vi "Test Bench v21 - TDMS.vi"() -> ()   [LabVIEW 2022 SP3]
doc: "Use this template to build a producer/consumer design pattern. Use this template when you need to execute a process, such as data analysis, when a data source, such as a triggered acquisition, produces data at an uneven rate and you need to execute the process when the data becomes available."
uses:
  WhiteNoise.ctl
  <vilib>/Utility/error.llb/DialogType.ctl
  <vilib>/Platform/TimedLoop/XDataNode/timing_clust.ctl
  <vilib>/Platform/TimedLoop/XDataNode/nitl_modes.ctl
  <vilib>/Platform/TimedLoop/XDataNode/wakeup.ctl
  <vilib>/DAQmx/write.llb/DAQmx Write (Analog Wfm 1Chan NSamp).vi
  <vilib>/DAQmx/read.llb/DAQmx Read (Analog Wfm 1Chan NSamp).vi
  <vilib>/DAQmx/miscellaneous.llb/DAQmx Fill In Error Info.vi
  <vilib>/measure/maspectr.llb/FFT Spectrum (Mag-Phase) for 1 Chan.vi
  <vilib>/platform/TimedLoop/XDataNode/XDataNode.xnode
  <vilib>/Platform/TimedLoop/XDataNode/XDNodeRunTimeDep.lvlib
  <vilib>/measure/NI_MAPro.lvlib
panel:
  out "error out":errorcluster
  in  "stop":bool
  out "Iteration Duration 3":i64
  in  "samples per channel":i32=41200
  in  "Folder to save file to":path=path "C:/Users/LAV-UFSC-2023/Documents/LAV-TCC/Dados-Experimentos/Dados-Bancada-LABVIEW"
  out "# pending insert":i32
  out "# pending remove":i32
  out "# elements in queue":i32
  out "Processor 2":i32=-2
  out "Iteration Duration":i64
  out "Processor":i32=-2
  out "Accelerometer":waveform(dbl)(graph)
  out "New file path":path
  in  "Log Data":bool=TRUE
  in  "view":T1={"dB On (F)"=FALSE, "unwrap phase (F)"=TRUE, "convert to degree (F)"=TRUE}
  out "FFT - Phase":cluster{"f0":dbl, "df":dbl, "phase":dbl[]}(graph)
  out "FFT - Magnitude":cluster{"f0":dbl, "df":dbl, "magnitude":dbl[]}(graph)
  out "Signal Output (V)":waveform(dbl)(graph)
  out "Iteration Duration 2":i64
  in  "Enable Output":bool=TRUE
  in  "Signal Output\nControl":enum32{"White Noise", "Harmonic"}(tab)
  in  "White Noise\nParameters":T3={"Seed"=0.0, "Standard Deviation"=2.0, "Reset"=FALSE, "Iterator"=1.0, "Lower Cut-Off"=5.0, "Upper Cut-Off"=350.0} {"Upper Cut-Off" min=5.0 max=350.0 step=10.0; "Lower Cut-Off" min=5.0 max=350.0 step=10.0; "Standard Deviation" min=0.001 max=3.0 step=0.05 format="%0.2p"}
  in  "Hamonic\nParameters":T4={"Waveform Type"=0, "Frequency (Hz)"=10.0, "Amplitude"=0.25} {"Frequency (Hz)" min=5.0 max=350.0 step=10.0 format="%0.2p"; "Waveform Type" items=["Sine Wave", "Triangle Wave", "Square Wave", "Sawtooth Wave"]; "Amplitude" min=0.001 max=0.3 step=0.05 format="%0.2p"}
  # "Debug Pannel"
  # "Filter"
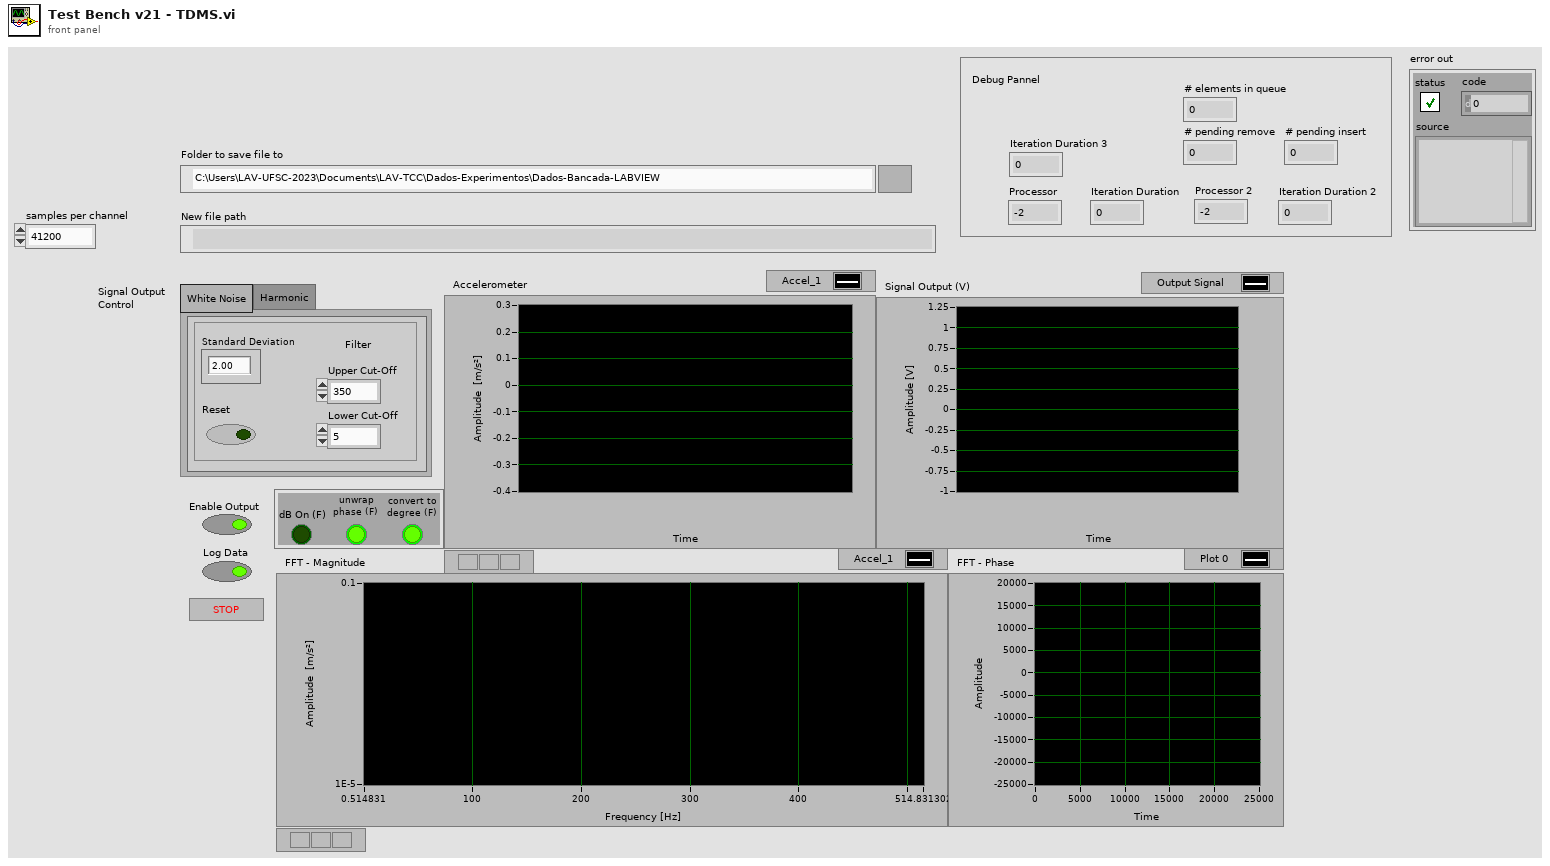
[diagram p1: front panel]
types:
  T1 = cluster{"dB On (F)":bool, "unwrap phase (F)":bool, "convert to degree (F)":bool}
  T2 = typedef "WhiteNoise.ctl" = dbl
  T3 = cluster{"Seed":T2, "Standard Deviation":dbl, "Reset":bool, "Iterator":dbl, "Lower Cut-Off":dbl, "Upper Cut-Off":dbl}
  T4 = cluster{"Waveform Type":u16, "Frequency (Hz)":dbl, "Amplitude":dbl}
  T5 = cluster{"FrameProperties":cluster{"Frame Duration":i64, "Actual Start [i]":i64}, "Accelerometer 1":waveform(dbl), "SignalOut":waveform(dbl)}
  T6 = typedef "XDNodeRunTimeDep.lvlib/timing_clust.ctl" = cluster{"Expected End [f-1]":u64, "Actual End [f-1]":u64, "Finished Late? [f-1]":bool, "Expected End [i-1]":u64, "Actual End [i-1]":u64, "Finished Late? [i-1]":bool, "Expected Start [i]":u64, "Actual Start [i]":u64, "Expected Start [f]":u64, "Actual Start [f]":u64, "Source Name":string, "Structure Name":string, "Period":i64, "Deadline":i64, "Offset":i64, "Start":i64, "Priority":i32, "Timeout":i32, "Mode":T7, "Wakeup Reason":T8, "Error":errorcluster, "Source Type":string, "Secondary Source Type":string, "Global End Time":u64, "Global Start Time":u64, "Frame Duration":u64, "Iteration Duration":u64, "Assigned CPU":i32, "I/O Scan Engine Mode":u32}
  T7 = typedef "XDNodeRunTimeDep.lvlib/nitl_modes.ctl" = enum32{"No Change", "Process missed periods, maintain original phase", "Discard missed periods, maintain original phase", "Process missed periods, ignore original phase", "Discard missed periods, ignore original phase"}
  T8 = typedef "XDNodeRunTimeDep.lvlib/wakeup.ctl" = enum32{"Normal", "Aborted", "Asynchronous wakeup", "Timing source error", "Timed loop error", "Timeout"}
  T9 = typedef "DialogType.ctl" = u16
  T10 = cluster{"Frame Duration":i64, "Actual Start [i]":i64}
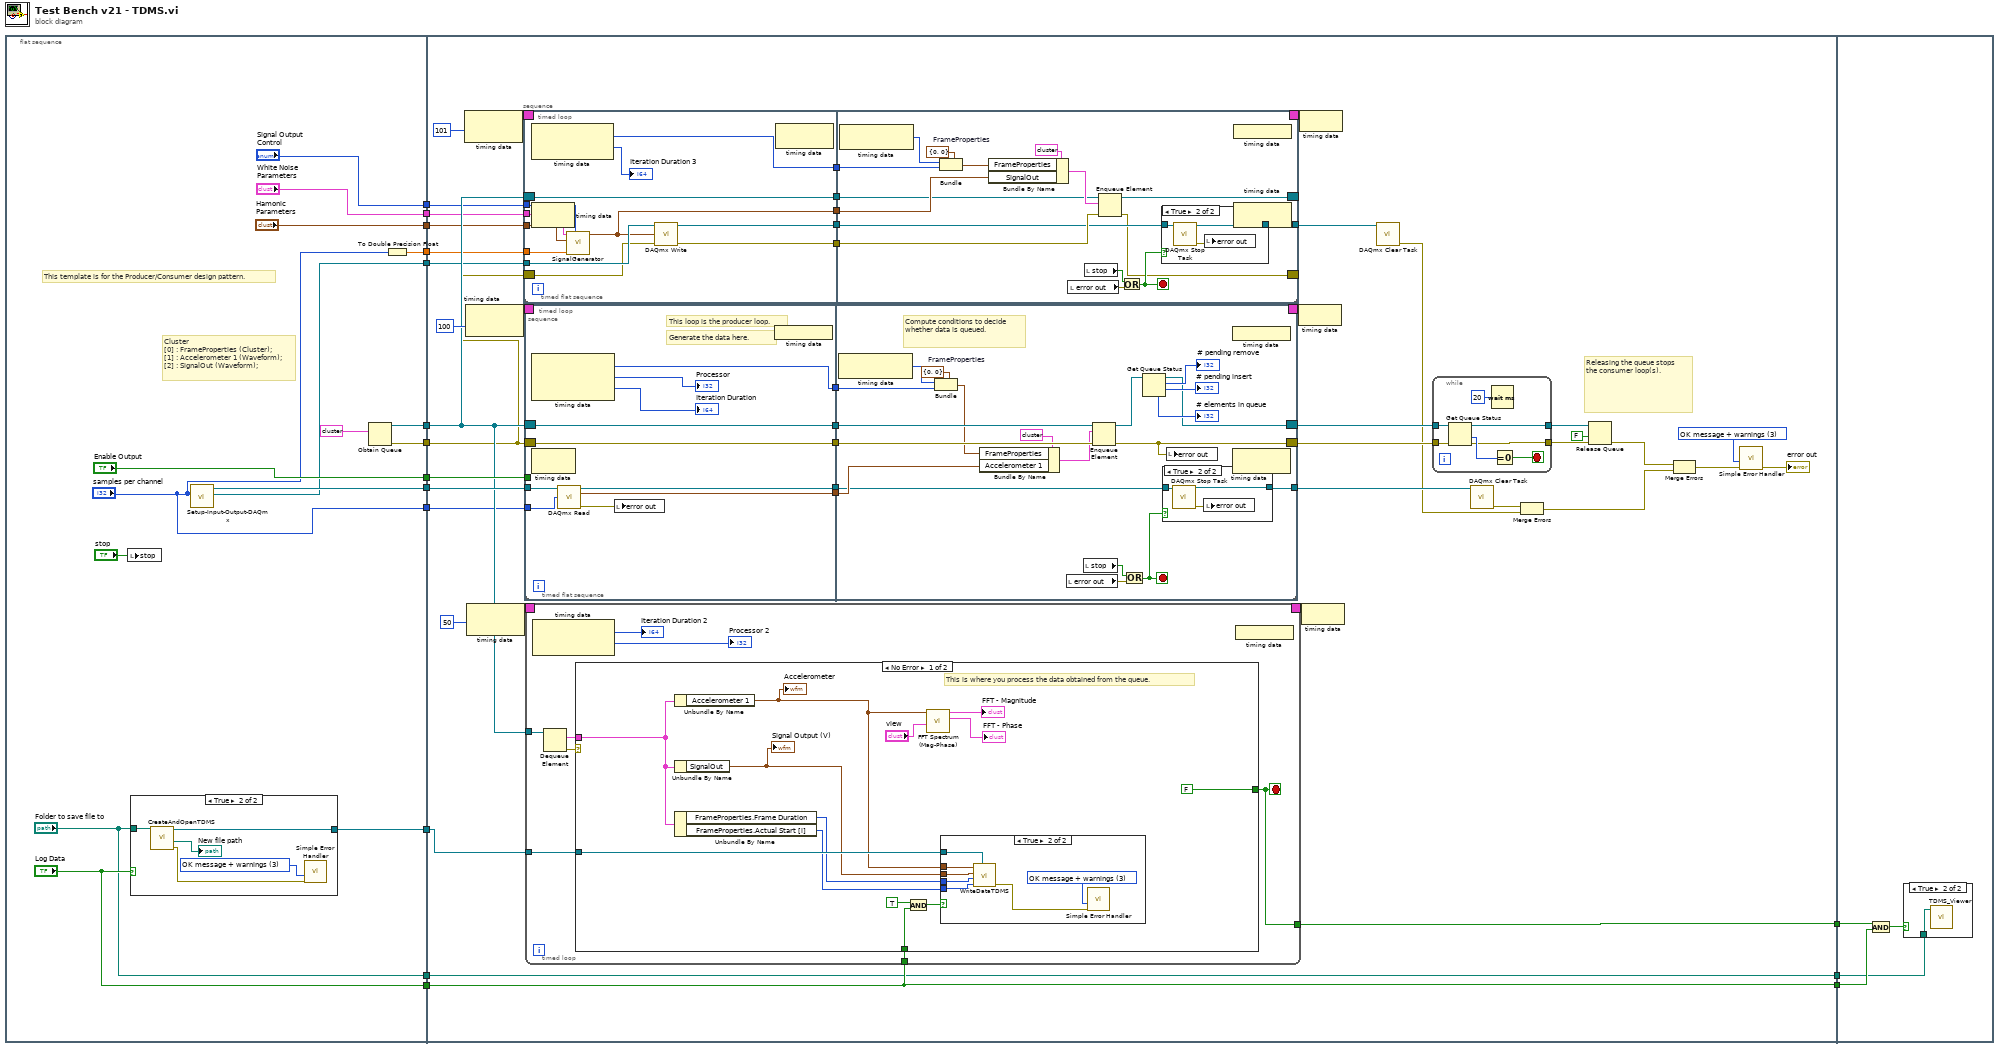
[diagram p0: block diagram]
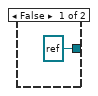
[diagram p2: hidden frame]
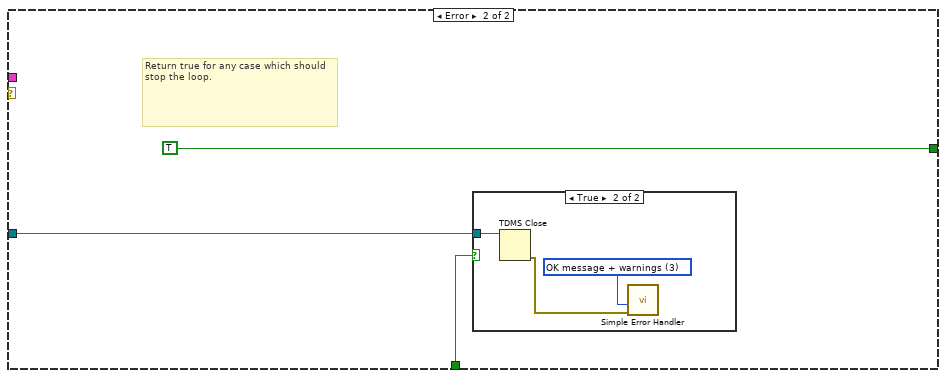
[diagram p5: hidden frame]
diagram:
  n1 = flat-sequence {
    tunnel: [w31] -> w16
    tunnel: [w30] -> w15
    tunnel: ["Log Data"] -> w14
    tunnel: ["Folder to save file to"] -> w10
    tunnel: ["Enable Output"] -> w9
    tunnel: [w25] -> w8
    tunnel: [w24] -> w7
    tunnel: ["samples per channel"] -> w6
    tunnel: [w23] -> w5
    tunnel: ["Signal Output\nControl"] -> w4
    tunnel: ["White Noise\nParameters"] -> w3
    tunnel: ["Hamonic\nParameters"] -> w2
    tunnel: [w19] -> w1
    tunnel: w16 -> [w69]
    tunnel: w15 -> [w66]
    tunnel: w14 -> [w64]
    tunnel: [w64] -> w13
    tunnel: [w63] -> w12
    tunnel: [w62] -> w11
    tunnel: w10 -> [w62]
    tunnel: w9 -> [w51]
    tunnel: w8 -> [w47]
    tunnel: w7 -> [w38]
    tunnel: w6 -> [w46]
    tunnel: w5 -> [w45]
    tunnel: w4 -> [w44]
    tunnel: w3 -> [w43]
    tunnel: w2 -> [w42]
    tunnel: w1 -> [w41]
    tunnel: w11 -> [w264]
    tunnel: w12 -> [w263]
    tunnel: w13 -> [w265]
    frame #0 {
      # "Cluster\n[0] : FrameProperties (Cluster);\n[1] : Accelerometer 1 (Waveform);\n[2] : SignalOut (Waveform);"
      # "This template is for the Producer/Consumer design pattern."
      n2 = local write "stop"("stop") -> ()
      n3 = case shown="True" "Log Data" {
        tunnel: [refnum<k34> refnum ("tdms file out") w34] -> w30
        tunnel: "Folder to save file to" -> [_ w33]
        frame False {
        }
        frame True {
          w36 = T9 3 items=["no dialog", "OK message", "continue or stop message", "OK message + warnings", "continue/stop + warnings"] ("type of dialog (OK msg:1)")
          n4 = call "CreateAndOpenTDMS.vi"("Folder to save file to"=w33) -> ("error out"=w37:errorcluster, "New file path"=→"New file path":path, "tdms file out"=w34:refnum<k34>)  [unwired: 8 in]
          n5 = call <vilib>:"Simple Error Handler.vi"("type of dialog (OK msg:1)"=w36, "error in (no error)"=w37) -> ()  [unwired: 3 in, 5 out]
        }
      }
      n6 = call "Setup-Input-Output-DAQmx.vi"("samples per channel"="samples per channel") -> ("Output task"=w23:refnum<k21>, "Input Task"=w31:refnum<k21>)  [unwired: 8 in, 1 out]
      n7 = Obtain Queue(element data type=T5 {"FrameProperties"={"Frame Duration"=0, "Actual Start [i]"=0}, "Accelerometer 1"={"t0"=timestamp(0 s since 1904-01-01), "dt"=1.0, "Y"=[]}, "SignalOut"={"t0"=timestamp(0 s since 1904-01-01), "dt"=1.0, "Y"=[]}} ("input cluster")) -> (queue out=w25:refnum<queue>, error out=w24:errorcluster)  [unwired: 4 in, 1 out]
      n8 = To Double Precision Float(number="samples per channel") -> (double precision float=w19:dbl)
    }
    frame #1 {
      w53 = T9 3 items=["no dialog", "OK message", "continue or stop message", "OK message + warnings", "continue/stop + warnings"] ("type of dialog (OK msg:1)")
      # "Releasing the queue stops the consumer loop(s)."
      n9 = node-c288(101 ("Priority")) -> (w50:T6)
      n10 = node-c288(100 ("Priority")) -> (w74:T6)
      n11 = node-c288(50 ("Priority")) -> (w72:T6)
      n12 = timed-loop {
        timing: w50 -> [_]
        timing-out: [_] -> w49
        shift-right: [w84] -> _
        shift-left: w47 -> [w79]
        tunnel: w45 -> [w83]
        tunnel: w44 -> [w82]
        tunnel: w43 -> [w81]
        tunnel: w42 -> [w80]
        tunnel: w41 -> [w78]
        tunnel: [w77] -> w39
        shift-right: [w76] -> _
        shift-left: w38 -> [w75]
        stop <- w119 stop-if-true
        n13 = timed-sequence {
          timing: _ -> [_]
          timing-out: _ -> [_]
          tunnel: [w99] -> w84
          tunnel: w83 -> [w98]
          tunnel: w82 -> [w97]
          tunnel: w81 -> [w96]
          tunnel: w80 -> [w95]
          tunnel: w79 -> [w91]
          tunnel: w78 -> [w90]
          tunnel: [w87] -> w77
          tunnel: [w86] -> w76
          tunnel: w75 -> [w85]
          n14 = timed-flat-sequence {
            tunnel: w98 -> [w111]
            tunnel: w97 -> [w110]
            tunnel: w96 -> [w109]
            tunnel: w95 -> [w108]
            tunnel: [w106] -> w94
            tunnel: [w105] -> w93
            tunnel: [w104] -> w92
            tunnel: w91 -> [w104]
            tunnel: w90 -> [w103]
            tunnel: [w102] -> w89
            tunnel: [w101] -> w88
            tunnel: w85 -> [w100]
            tunnel: [w123] -> w99
            tunnel: w94 -> [w126]
            tunnel: w93 -> [w125]
            tunnel: w92 -> [w124]
            tunnel: w89 -> [w122]
            tunnel: w88 -> [w117]
            tunnel: [w118] -> w87
            tunnel: [w116] -> w86
            frame #0 {
              n15 = node-c288() -> (w106:i64, →"Iteration Duration 3":i64)  [unwired: 1 in]
              n16 = call "SignalGenerator.vi"("Signal Output\nControl"=w110, "#s"=w103, "Hamonic\nParameters"=w108, "White Noise\nParameters"=w109) -> ("Signal Out"=w105:waveform(dbl))  [unwired: 7 in]
              n17 = call-poly <vilib>:"DAQmx Write.vi"("task/channels in"=w111, "data"=w105, "error in"=w100) -> ("task out"=w101:refnum<k21>, "error out"=w102:errorcluster)  [unwired: 10 in, 1 out]
              n18 = node-c288() -> ()  [unwired: 1 in, 1 out]
            }
            frame #1 {
              w129 = T10 {"Frame Duration"=0, "Actual Start [i]"=0}  # FrameProperties
              n19 = node-c288() -> (w127:i64)  [unwired: 1 in]
              n20 = Bundle(cluster=w129, "Frame Duration"=w127, "Actual Start [i]"=w126) -> (w130:T10)
              n21 = Bundle By Name(cluster=T5 {"FrameProperties"={"Frame Duration"=0, "Actual Start [i]"=0}, "Accelerometer 1"={"t0"=timestamp(0 s since 1904-01-01), "dt"=1.0, "Y"=[]}, "SignalOut"={"t0"=timestamp(0 s since 1904-01-01), "dt"=1.0, "Y"=[]}} ("input cluster"), "FrameProperties"=w130, "SignalOut"=w125) -> (w131:T5)
              n22 = local read "error out"() -> (w121:errorcluster)
              n23 = local read "stop"() -> (w120:bool)
              n24 = Enqueue Element(queue=w124, element=w131, error in (no error)=w122) -> (queue out=w123:refnum<queue>, error out=w116:errorcluster)  [unwired: 1 in, 1 out]
              n25 = Or(x=w120, y=w121) -> (x .or. y?=w119:bool)
              n26 = case shown="True" w119 {
                tunnel: [w132 w135] -> w118
                tunnel: w117 -> [w132 w134]
                frame False {
                }
                frame True {
                  n27 = call <vilib>:"DAQmx Stop Task.vi"("task/channels in"=w134) -> ("task out"=w135:refnum<k21>, "error out"=w133:errorcluster)  [unwired: 13 in]
                  n28 = local write "error out"(w133) -> ()
                }
              }
              n29 = node-c288() -> ()  [unwired: 1 out]
            }
          }
        }
        n30 = node-c288() -> ()  [unwired: 1 in, 1 out]
        n31 = node-c288() -> ()  [unwired: 1 in, 1 out]
      }
      n32 = timed-loop {
        shift-right: [w196] -> w61
        shift-left: w38 -> [w200]
        shift-right: [w198] -> w65
        shift-left: w47 -> [w199]
        tunnel: [w197] -> w68
        tunnel: w69 -> [w201]
        timing: w74 -> [_]
        timing-out: [_] -> w73
        tunnel: w51 -> [w195]
        tunnel: w46 -> [w194]
        stop <- w230 stop-if-true
        n33 = timed-sequence {
          timing: _ -> [_]
          timing-out: _ -> [_]
          tunnel: w201 -> [w214]
          tunnel: w200 -> [w213]
          tunnel: w199 -> [w212]
          tunnel: [w211] -> w198
          tunnel: [w205] -> w197
          tunnel: [w204] -> w196
          tunnel: w195 -> [w203]
          tunnel: w194 -> [w202]
          n34 = timed-flat-sequence {
            tunnel: w214 -> [w218]
            tunnel: w213 -> [w224]
            tunnel: w212 -> [w223]
            tunnel: [w219] -> w210
            tunnel: [w224] -> w209
            tunnel: [w223] -> w208
            tunnel: [w222] -> w207
            tunnel: [w217] -> w206
            tunnel: w203 -> [_]
            tunnel: w202 -> [w216]
            tunnel: [w236] -> w211
            tunnel: w210 -> [w235]
            tunnel: w209 -> [w249]
            tunnel: w208 -> [w248]
            tunnel: w207 -> [w246]
            tunnel: w206 -> [w245]
            tunnel: [w234] -> w205
            tunnel: [w233] -> w204
            frame #0 {
              # "Generate the data here."
              # "This loop is the producer loop."
              n35 = node-c288() -> (w222:i64, →"Processor":i32, →"Iteration Duration":i64)  [unwired: 1 in]
              n36 = call-poly <vilib>:"DAQmx Read.vi"("task/channels in"=w218, "number of samples per channel"=w216) -> ("task out"=w219:refnum<k21>, "data"=w217:waveform(dbl), "error out"=w215:errorcluster)  [unwired: 11 in]
              n37 = local write "error out"(w215) -> ()
              n38 = node-c288() -> ()  [unwired: 1 out]
            }
            frame #1 {
              w242 = T10 {"Frame Duration"=0, "Actual Start [i]"=0}  # FrameProperties
              # "Compute conditions to decide whether data is queued."
              n39 = node-c288() -> (w247:i64)  [unwired: 1 in]
              n40 = Bundle(cluster=w242, "Frame Duration"=w247, "Actual Start [i]"=w246) -> (w243:T10)
              n41 = Bundle By Name(cluster=T5 {"FrameProperties"={"Frame Duration"=0, "Actual Start [i]"=0}, "Accelerometer 1"={"t0"=timestamp(0 s since 1904-01-01), "dt"=1.0, "Y"=[]}, "SignalOut"={"t0"=timestamp(0 s since 1904-01-01), "dt"=1.0, "Y"=[]}} ("input cluster"), "FrameProperties"=w243, "Accelerometer 1"=w245) -> (w244:T5)
              n42 = local read "error out"() -> (w232:errorcluster)
              n43 = local read "stop"() -> (w231:bool)
              n44 = Enqueue Element(queue=w248, element=w244, error in (no error)=w249) -> (queue out=w237:refnum<queue>, error out=w233:errorcluster)  [unwired: 1 in, 1 out]
              n45 = Or(x=w231, y=w232) -> (x .or. y?=w230:bool)
              n46 = Get Queue Status(queue=w237) -> (queue out=w236:refnum<queue>, # pending remove=→"# pending remove":i32, # pending insert=→"# pending insert":i32, # elements in queue=→"# elements in queue":i32)  [unwired: 2 in, 4 out]
              n47 = case shown="True" w230 {
                tunnel: [w250 w253] -> w234
                tunnel: w235 -> [w250 w252]
                frame False {
                }
                frame True {
                  n48 = call <vilib>:"DAQmx Stop Task.vi"("task/channels in"=w252) -> ("task out"=w253:refnum<k21>, "error out"=w251:errorcluster)  [unwired: 13 in]
                  n49 = local write "error out"(w251) -> ()
                }
              }
              n50 = local write "error out"(w233) -> ()
              n51 = node-c288() -> ()  [unwired: 1 out]
            }
          }
        }
        n52 = node-c288() -> ()  [unwired: 1 in, 1 out]
        n53 = node-c288() -> ()  [unwired: 1 in, 1 out]
      }
      n54 = timed-loop {
        tunnel: w47 -> [w159]
        timing: w72 -> [_]
        timing-out: [_] -> w71
        tunnel: w64 -> [w154]
        tunnel: [w152] -> w63
        tunnel: w66 -> [w155]
        stop <- w152 stop-if-true
        n55 = node-c288() -> (→"Iteration Duration 2":i64, →"Processor 2":i32)  [unwired: 1 in]
        n56 = Dequeue Element(queue=w159) -> (element=w157:T5, error out=w158:errorcluster)  [unwired: 2 in, 2 out]
        n57 = case shown="No Error" w158 {
          tunnel: w157 -> [w172 _]
          tunnel: [FALSE TRUE] -> w152
          tunnel: w155 -> [w173 w184]
          tunnel: w154 -> [w165 w185]
          frame No Error {
            # "This is where you process the data obtained from the queue."
            n58 = Unbundle By Name(w172) -> ("Accelerometer 1"=w171:waveform(dbl))
            "Accelerometer" <- w171
            n59 = Unbundle By Name(w172) -> ("SignalOut"=w170:waveform(dbl))
            "Signal Output (V)" <- w170
            n60 = Unbundle By Name(w172) -> ("FrameProperties.Frame Duration"=w169:i64, "FrameProperties.Actual Start [i]"=w168:i64)
            n61 = And(x=TRUE, y=w165) -> (x .and. y?=w166:bool)
            n62 = call-poly <vilib>:"FFT Spectrum (Mag-Phase).vi"("view"="view", "time signal"=w171) -> ("phase"=→"FFT - Phase":cluster{"f0":dbl, "df":dbl, "phase":dbl[]}, "magnitude"=→"FFT - Magnitude":cluster{"f0":dbl, "df":dbl, "magnitude":dbl[]})  [unwired: 5 in, 3 out]
            n63 = case shown="True" w166 {
              tunnel: w173 -> [_ w183]
              tunnel: w171 -> [_ w182]
              tunnel: w170 -> [_ w181]
              tunnel: w169 -> [_ w180]
              tunnel: w168 -> [_ w179]
              frame False {
              }
              frame True {
                w178 = T9 3 items=["no dialog", "OK message", "continue or stop message", "OK message + warnings", "continue/stop + warnings"] ("type of dialog (OK msg:1)")
                n64 = call "WriteDataTDMS.vi"("tdms file"=w183, "ActualStart[f]"=w179, "TimeInterval"=w180, "SignalOut"=w181, "Accel."=w182) -> ("error out"=w177:errorcluster)  [unwired: 5 in, 1 out]
                n65 = call <vilib>:"Simple Error Handler.vi"("type of dialog (OK msg:1)"=w178, "error in (no error)"=w177) -> ()  [unwired: 3 in, 5 out]
              }
            }
          }
          frame Error {
            # "Return true for any case which should stop the loop."
            n66 = case shown="True" w185 {
              tunnel: w184 -> [_ w188]
              frame False {
              }
              frame True {
                w189 = T9 3 items=["no dialog", "OK message", "continue or stop message", "OK message + warnings", "continue/stop + warnings"] ("type of dialog (OK msg:1)")
                n67 = TDMS Close(11:w188) -> (0:w187:errorcluster)  [unwired: 1 in, 1 out]
                n68 = call <vilib>:"Simple Error Handler.vi"("type of dialog (OK msg:1)"=w189, "error in (no error)"=w187) -> ()  [unwired: 3 in, 5 out]
              }
            }
          }
        }
        n69 = node-c288() -> ()  [unwired: 1 out]
      }
      n70 = node-c288(w73) -> ()
      n71 = node-c288(w49) -> ()
      n72 = node-c288(w71) -> ()
      n73 = call <vilib>:"DAQmx Clear Task.vi"("task in"=w39) -> ("error out"=w57:errorcluster)  [unwired: 14 in]
      n74 = while {
        tunnel: w61 -> [w151]
        tunnel: w65 -> [w150]
        tunnel: [w147] -> w60
        tunnel: [w146] -> w59
        stop <- w148 stop-if-true
        n75 = Get Queue Status(queue=w150, error in (no error)=w151) -> (queue out=w146:refnum<queue>, # pending insert=w149:i32, error out=w147:errorcluster)  [unwired: 1 in, 5 out]
        n76 = Wait (ms)(milliseconds to wait=u32 20) -> ()  [unwired: 1 out]
        n77 = Equal To 0?(x=w149) -> (x = 0?=w148:bool)
      }
      n78 = call <vilib>:"DAQmx Clear Task.vi"("task in"=w68) -> ("error out"=w58:errorcluster)  [unwired: 14 in]
      n79 = Merge Errors(w58, w57) -> (w54:errorcluster)
      n80 = Release Queue(queue=w59, force destroy? (F)=FALSE, error in (no error)=w60) -> (error out=w55:errorcluster)  [unwired: 2 out]
      n81 = Merge Errors(w55, w54) -> (w56:errorcluster)
      n82 = call <vilib>:"Simple Error Handler.vi"("type of dialog (OK msg:1)"=w53, "error in (no error)"=w56) -> ("error out"=→"error out":errorcluster)  [unwired: 3 in, 4 out]
    }
    frame #2 {
      n83 = And(x=w263, y=w265) -> (x .and. y?=w266:bool)
      n84 = case shown="True" w266 {
        tunnel: w264 -> [_ w267]
        frame False {
        }
        frame True {
          n85 = call "TDMS_Viewer.vi"("Data Directory"=w267) -> ()  [unwired: 11 in]
        }
      }
    }
  }
